vi "Data Type Selector Popup.vi"(8 "error in (no error)":errorcluster, 11 "Data Type Selector in":refnum<class "Data Type Selector.lvclass">) -> ()   [LabVIEW 2018, in "Data Type Selector.lvclass"]
uses:
  Data Type Selector.lvclass
  Data Type Selector.lvclass/Data Type Selector.ctl
  <vilib>/MGI/Panel Manager/Panel/Panel/Panel.lvclass
  Data Type Classes/Generic/Generic Data Type.lvclass
panel:
  in  "Data Type Selector":string(combo)
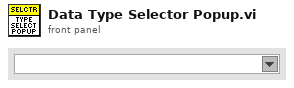
[diagram p1: front panel]
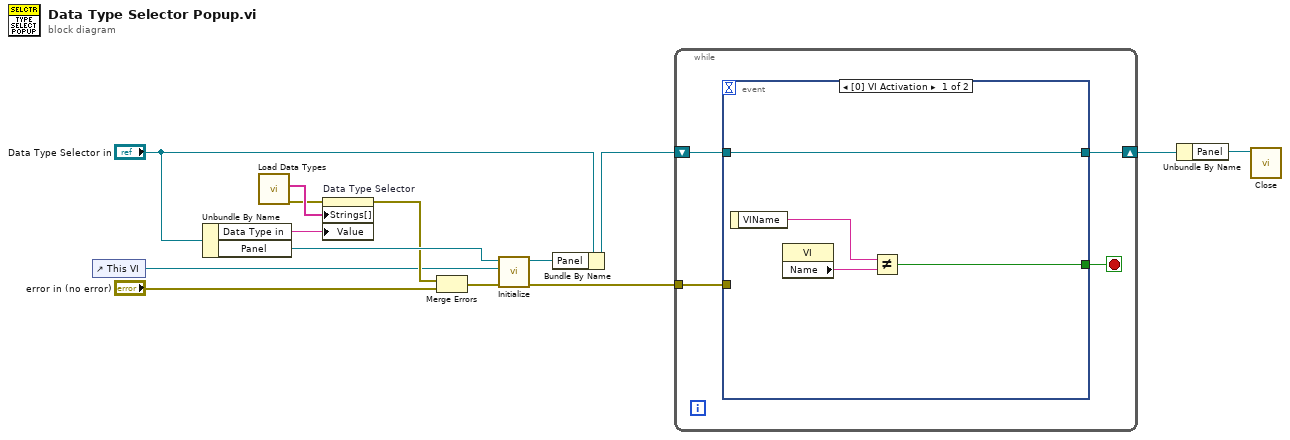
[diagram p0: block diagram]
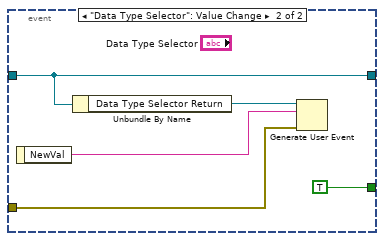
[diagram p2: hidden frame]
diagram:
  n1 = control-ref of="This VI"() -> (w9:refnum<vi>)
  n2 = Unbundle By Name("Data Type Selector in") -> ("Data Type in"=w7:string, "Panel"=w14:refnum<class "Panel.lvclass">)
  n3 = call "Load Data Types.vi"() -> ("error out"=w5:errorcluster, "Data Type Names"=w6:string[])  [unwired: 9 in, 1 out]
  n4 = property on="Data Type Selector" class="CmbBox"(error in=w5, "Strings[]"=w6, "Value"=w7) -> (error out=w13:errorcluster)  [unwired: 1 in, 1 out]
  n5 = Merge Errors(w13, "error in (no error)") -> (w4:errorcluster)
  n6 = call <vilib>:"Initialize.vi"("error in (no error)"=w4, "VI Refnum"=w9, "Panel In"=w14) -> ("error out"=w10:errorcluster, "Panel Out"=w3:refnum<class "Panel.lvclass">)  [unwired: 6 in, 1 out]
  n7 = Bundle By Name(cluster="Data Type Selector in", "Panel"=w3) -> (w1:refnum<class "Data Type Selector.lvclass">)
  n8 = while {
    shift-right: [w16] -> w12
    shift-left: w1 -> [w17]
    tunnel: w10 -> [w15]
    stop <- w18 stop-if-true
    n9 = event shown="[0] VI Activation" {
      selector: _ -> [_ _]
      dyn-events: _ -> [_ _]
      timeout: _ -> [_ _]
      tunnel: [w20 TRUE] -> w18
      tunnel: w17 -> [w19 w27]
      tunnel: [w19 w27] -> w16
      tunnel: w15 -> [_ w25]
      event VI Activation {
        n10 = event-data() -> ("VIName"=w22:string)  [unwired: 1 in]
        n11 = property class="VI"() -> ("Name"=w21:string)  [unwired: 2 in, 2 out]
        n12 = Not Equal?(x=w22, y=w21) -> (x != y?=w20:bool)
      }
      event "Data Type Selector": Value Change {
        n13 = event-data() -> ("NewVal"=w24:string)  [unwired: 1 in]
        n14 = Unbundle By Name(w27) -> ("Data Type Selector Return"=w26:refnum<user-event>)
        n15 = Generate User Event(user event=w26, event data cluster=w24, error in=w25) -> ()  [unwired: 1 in, 2 out]
      }
    }
  }
  n16 = Unbundle By Name(w12) -> ("Panel"=w11:refnum<class "Panel.lvclass">)
  n17 = call-dynamic "Close.vi"("Panel In"=w11) -> ()  [unwired: 10 in, 1 out]
